vi "Trigger Detector (Complex Spectra).vi"(0 "complex spectra":cluster{"f0":dbl, "df":dbl, "vectors":cdb[]}[](array[cluster]), 1 "reset? (F)":bool, 5 "triggers definition":T3(array[cluster]), 9 "data timestamp":timestamp, 11 "error in (no error)":errorcluster) -> (4 "triggers":T2(array[cluster]), 6 "actual trigger state":T1[](array[typedef]), 15 "error out":errorcluster)   [LabVIEW 2014, in "NI_EP_Power Quality.lvlib"]
doc: "Detects crossing of limits for the measurement that you specify and returns triggers if occur.\n\nThis VI supports measuring single-line and multiple-line systems except the DBL instance. Use the DBL instance to measure one channel on one line at one time."
uses:
  <vilib>/addons/Electrical Power/PQ/NI_EP_Power Quality.lvlib
  <vilib>/addons/Electrical Power/PQ/Common/Controls/ep_Trigger State.ctl
  <vilib>/addons/Electrical Power/PQ/Triggers/subVIs/ep_Trigger Definition.ctl
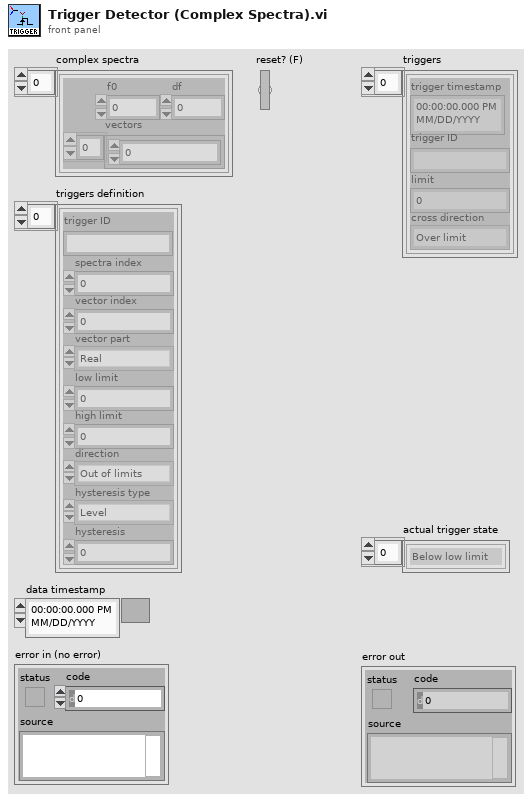
[diagram p1: front panel]
types:
  T1 = typedef "NI_EP_Power Quality.lvlib/ep_Trigger State.ctl" = enum16{"Below low limit", "In the limits", "Over high limit"}
  T2 = cluster{"trigger timestamp":timestamp, "trigger ID":string, "limit":dbl, "cross direction":enum16{"Over limit", "Below limit"}}[]
  T3 = cluster{"trigger ID":string, "spectra index":u32, "vector index":u32, "vector part":enum16{"Real", "Imaginary", "R", "Theta"}, "low limit":dbl, "high limit":dbl, "direction":enum16{"Out of limits", "Back to limits", "Both"}, "hysteresis type":enum16{"Level", "Time"}, "hysteresis":dbl}[]
  T4 = cluster{"trigger time":timestamp, "trigger unique id":string, "limit":dbl, "cross direction":enum16{"Over limit", "Below limit"}}[]
  T5 = typedef "NI_EP_Power Quality.lvlib/ep_Trigger Definition.ctl" = cluster{"trigger ID":string, "low limit":dbl, "high limit":dbl, "direction":enum16{"Out of limits", "Back to limits", "Both"}, "hysteresis type":enum16{"Level", "Time"}, "hysteresis":dbl}
  T6 = cluster{"Lo in progr.":bool, "Hi in progr.":bool, "Lo trig. time":timestamp, "Hi trig. time":timestamp}[]
  T7 = enum16{"Out of limits", "Back to limits", "Both"}
  T8 = cluster{"Lo in progr.":bool, "Lo in progr.":bool, "data timestamp":timestamp, "data timestamp":timestamp}
  T9 = cluster{"Lo in progr.":bool, "Hi in progr.":bool, "Lo trig. time":timestamp, "Hi trig. time":timestamp}
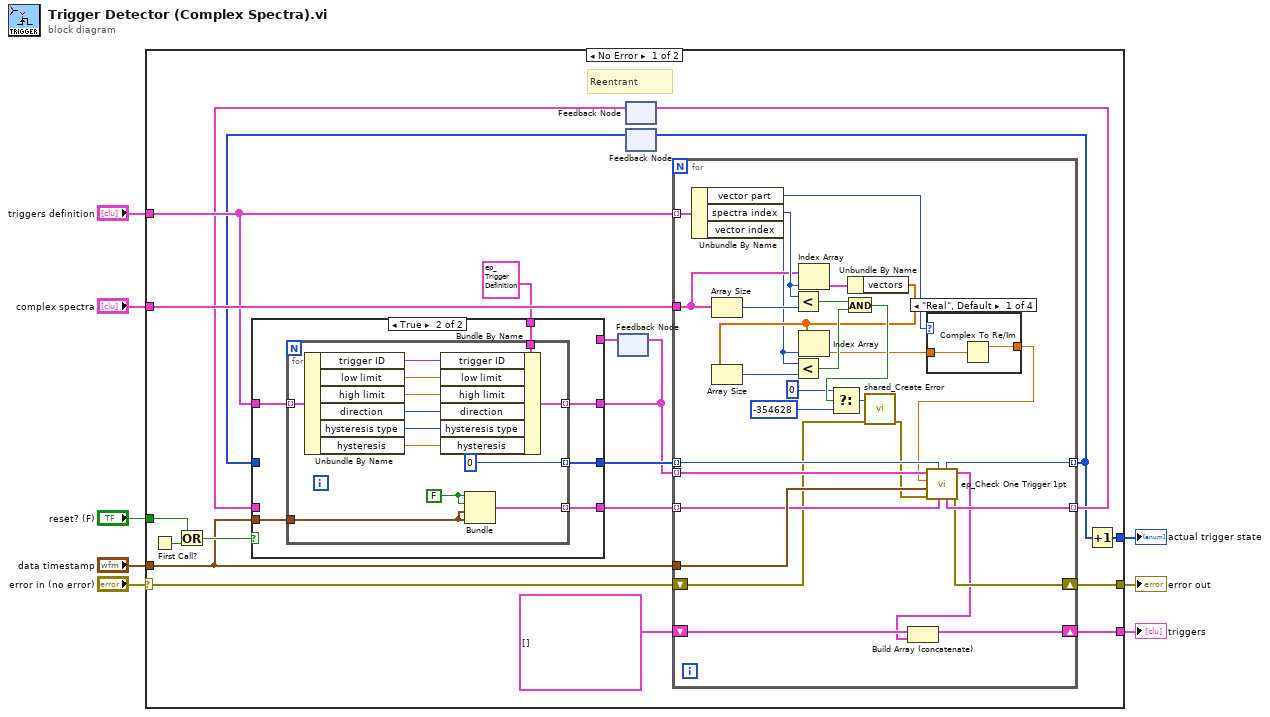
[diagram p0: block diagram]
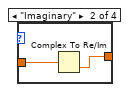
[diagram p3: hidden frame]
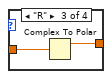
[diagram p4: hidden frame]
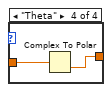
[diagram p5: hidden frame]
diagram:
  n1 = case shown="No Error" "error in (no error)" {
    selector: "error in (no error)" -> [w12 w88]
    tunnel: "complex spectra" -> [w28 _]
    tunnel: "reset? (F)" -> [w26 _]
    tunnel: "triggers definition" -> [w24 _]
    tunnel: [w14 _] -> w7
    tunnel: "data timestamp" -> [w13 _]
    tunnel: [w11 w88] -> w8
    tunnel: [w9 _] -> w1
    frame No Error {
      # "Reentrant"
      n2 = First Call?() -> (First Call?: T/F=w27:bool)
      n3 = Or(x=w26, y=w27) -> (x .or. y?=w25:bool)
      n4 = feedback #1() -> (w17:T5[])  [unwired: 1 in]
      n5 = feedback #2() -> (w18:T6)  [unwired: 1 in]
      n6 = feedback #3() -> (w20:i8[])  [unwired: 1 in]
      n7 = case shown="True" w25 {
        tunnel: w24 -> [_ w37]
        tunnel: [w29 w36] -> w16
        tunnel: T5 {"trigger ID"="", "low limit"=0.0, "high limit"=0.0, "direction"=enum."Out of limits", "hysteresis type"=enum."Level", "hysteresis"=0.0} ("trigger definition") -> [_ w35]
        tunnel: [w31 w34] -> w22
        tunnel: [w30 w33] -> w21
        tunnel: w20 -> [w30 _]
        tunnel: w18 -> [w31 _]
        tunnel: w17 -> [w29 _]
        tunnel: w13 -> [_ w32]
        frame False {
        }
        frame True {
          n8 = for {
            tunnel: w37 -> [w46] mode=indexing
            tunnel: [w45] -> w36 mode=indexing
            tunnel: w35 -> [w44]
            tunnel: [w40] -> w34 mode=indexing
            tunnel: [i8 0] -> w33 mode=indexing
            tunnel: w32 -> [w41]
            w42 = FALSE ("Lo in progr.")
            n9 = Unbundle By Name(w46) -> ("trigger ID"=w49:string, "low limit"=w39:dbl, "high limit"=w38:dbl, "direction"=w48:T7, "hysteresis type"=w47:enum16{"Level", "Time"}, "hysteresis"=w50:dbl)
            n10 = Bundle By Name(cluster=w44, "trigger ID"=w49, "low limit"=w39, "high limit"=w38, "direction"=w48, "hysteresis type"=w47, "hysteresis"=w50) -> (w45:T5)
            n11 = Bundle("Lo in progr."=w42, "Lo in progr."=w42, "data timestamp"=w41, "data timestamp"=w41) -> (w40:T8)  [unwired: 1 in]
          }
        }
      }
      n12 = feedback-in #1(w16) -> ()
      n13 = for {
        tunnel: w13 -> [w74]
        tunnel: w24 -> [w72] mode=indexing
        tunnel: w28 -> [w62]
        tunnel: w22 -> [w71] mode=indexing
        tunnel: w21 -> [w76] mode=indexing
        tunnel: [w75] -> w10 mode=indexing
        tunnel: [w73] -> w19 mode=indexing
        tunnel: w16 -> [w79] mode=indexing
        shift-right: [w78] -> w14
        shift-left: T4 [] -> [w77]
        shift-right: [w70] -> w11
        shift-left: w12 -> [w52]
        n14 = Unbundle By Name(w72) -> ("vector part"=w57:enum16{"Real", "Imaginary", "R", "Theta"}, "spectra index"=w63:u32, "vector index"=w59:u32)
        n15 = Array Size(array=w62) -> (size(s)=w67:i32)
        n16 = Less?(x=w63, y=w67) -> (x < y?=w66:bool)
        n17 = Index Array(array=w62, index=w63) -> (element=w61:cluster{"f0":dbl, "df":dbl, "vectors":cdb[]})
        n18 = Unbundle By Name(w61) -> ("vectors"=w60:cdb[])
        n19 = Array Size(array=w60) -> (size(s)=w69:i32)
        n20 = Less?(x=w59, y=w69) -> (x < y?=w65:bool)
        n21 = Index Array(array=w60, index=w59) -> (element=w58:cdb)
        n22 = And(x=w66, y=w65) -> (x .and. y?=w64:bool)
        n23 = Select(t=0 ("error code (0)"), s=w64, f=-354628 ("error code (0)")) -> (s? t:f=w53:i32)
        n24 = call <vilib>:"shared_Create Error.vi"("error in (no error)"=w52, "error code (0)"=w53) -> ("error out"=w51:errorcluster)  [unwired: 9 in]
        n25 = case shown="\"Real\", Default" w57 {
          tunnel: w58 -> [w81 w83 w85 w87]
          tunnel: [w80 w82 w84 w86] -> w56
          frame "Real", Default {
            n26 = Complex To Re/Im(x + iy=w81) -> (x=w80:dbl)  [unwired: 1 out]
          }
          frame "Imaginary" {
            n27 = Complex To Re/Im(x + iy=w83) -> (y=w82:dbl)  [unwired: 1 out]
          }
          frame "R" {
            n28 = Complex To Polar(r * e^(i*theta)=w85) -> (r=w84:dbl)  [unwired: 1 out]
          }
          frame "Theta" {
            n29 = Complex To Polar(r * e^(i*theta)=w87) -> (theta=w86:dbl)  [unwired: 1 out]
          }
        }
        n30 = call <vilib>:"ep_Check One Trigger 1pt.vi"("trig. local in"=w71, "prev. state in"=w76, "error in (no error)"=w51, "data time stamp"=w74, "value in"=w56, "trigger definition"=w79) -> ("error out"=w70:errorcluster, "triggers list"=w68:T4, "trig. local out"=w73:T9, "state out"=w75:i8)  [unwired: 2 in]
        n31 = Build Array (concatenate)(w77, w68) -> (w78:T4)
      }
      n32 = feedback-in #2(w19) -> ()
      n33 = feedback-in #3(w10) -> ()
      n34 = Increment(x=w10) -> (x+1=w9:i8[])
    }
    frame Error {
    }
  }
  "error out" <- w8
  "triggers" <- w7
  "actual trigger state" <- w1
